vi "Disable.vi"(8 "error in (no error)":errorcluster, 11 "PacificPowerSource in":refnum<class "PacificPowerSource.lvclass">) -> (0 "error out":errorcluster, 3 "PacificPowerSource out":refnum<class "PacificPowerSource.lvclass">)   [LabVIEW 2018, in "AcPwrPlugins.lvlib" / "PacificPowerSource.lvclass"]
doc: "This VI disables the output by opening the output switch."
uses:
  PacificPowerSource.lvclass
  <instrlib>/Pacific Power UPC Series/Pacific Power UPC Series.lvlib
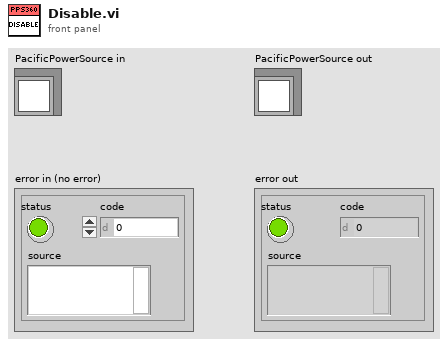
[diagram p1: front panel]
types:
  T1 = typedef "AcPwrPlugins.lvlib/PacificPowerSource.lvclass/Modules.ctl" = cluster{"Handle":string, "Connected":bool, "Clear Device (F)":bool, "btnIdQuery":bool, "btnReset":bool, "Program #":cluster{"Phase B (Degrees)":i32, "Waveform A (1: Sine)":i32, "Voltage Level (Va)":dbl, "Program Number (0)":i32, "Voltage Level (Vb) ":dbl, "Form (3: Three)":u16, "Coupling  (0: Direct)":u16, "Frequency (45Hz)":dbl, "Current Limit (40A)":dbl, "Phase C (Degrees)":i32, "Voltage Level (Vc)":dbl, "Waveform B (1: Sine)":i32, "Waveform C (1: Sine)":i32}[], "Impedance Parameters (off, 0.00)":cluster{"State":bool, "Impedance":dbl}, "Transient Execution (F)":bool, "OutputEnabled":bool, "Source Range":cluster{"Frequency Minimum (45 Hz)":dbl, "Frequency Maximum (1200 Hz)":dbl, "Voltage Maximum (V)":dbl, "Voltage Minimum (V)":dbl, "Range Control (0: Auto)":u16, "Initial Voltage (0V)":u16, "Frequency Range (600Hz)":u16}, "Port Type":enum16{"GPIB", "Serial"}}[]
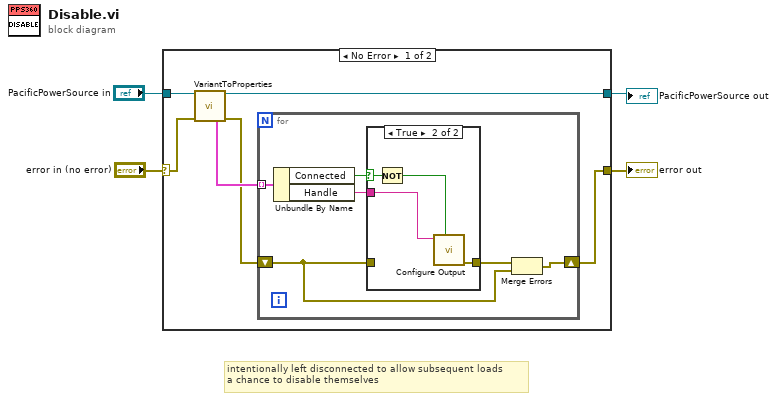
[diagram p0: block diagram]
diagram:
  # "intentionally left disconnected to allow subsequent loads\na chance to disable themselves"
  n1 = case shown="No Error" "error in (no error)" {
    selector: "error in (no error)" -> [w6 w23]
    tunnel: [w10 w23] -> w1
    tunnel: [w7 w22] -> w2
    tunnel: "PacificPowerSource in" -> [w5 w22]
    frame No Error {
      n2 = call "VariantToProperties.vi"("PacificPowerSource in"=w5, "error in (no error)"=w6) -> ("PacificPowerSource out"=w7:refnum<class "PacificPowerSource.lvclass">, "Modules"=w9:T1, "error out"=w8:errorcluster)  [unwired: 7 in, 4 out]
      n3 = for {
        tunnel: w9 -> [w16] mode=indexing
        shift-right: [w12] -> w10
        shift-left: w8 -> [w11]
        n4 = Unbundle By Name(w16) -> ("Connected"=w14:bool, "Handle"=w15:string)
        n5 = case shown="True" w14 {
          selector: w14 -> [_ w18]
          tunnel: w11 -> [w17 _]
          tunnel: [w17 w21] -> w13
          tunnel: w15 -> [_ w20]
          frame False {
          }
          frame True {
            n6 = Not(x=w18) -> (.not. x?=w19:bool)
            n7 = call <instrlib>:"Configure Output.vi"("Enable Output (T: Enable)"=w19, "VISA resource name"=w20) -> ("error out"=w21:errorcluster)  [unwired: 8 in, 1 out]
          }
        }
        n8 = Merge Errors(w13, w11) -> (w12:errorcluster)
      }
    }
    frame Error {
    }
  }
  "error out" <- w1
  "PacificPowerSource out" <- w2
